vi "solar_voy Set VI Control.vi"(8 "error in (no error)":errorcluster, 11 "VI_SET_CONTROL":T1) -> (0 "error out":errorcluster)   [LabVIEW 2018]
doc: "This sets a VI control value by VI and Control name. The Value must be the LabVIEW native data type."
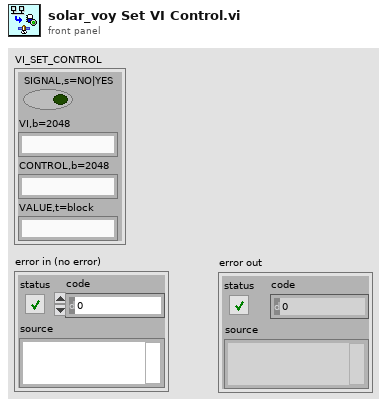
[diagram p1: front panel]
types:
  T1 = cluster{"SIGNAL,s=NO|YES":bool, "VI,b=2048":string, "CONTROL,b=2048":string, "VALUE,t=block":string}
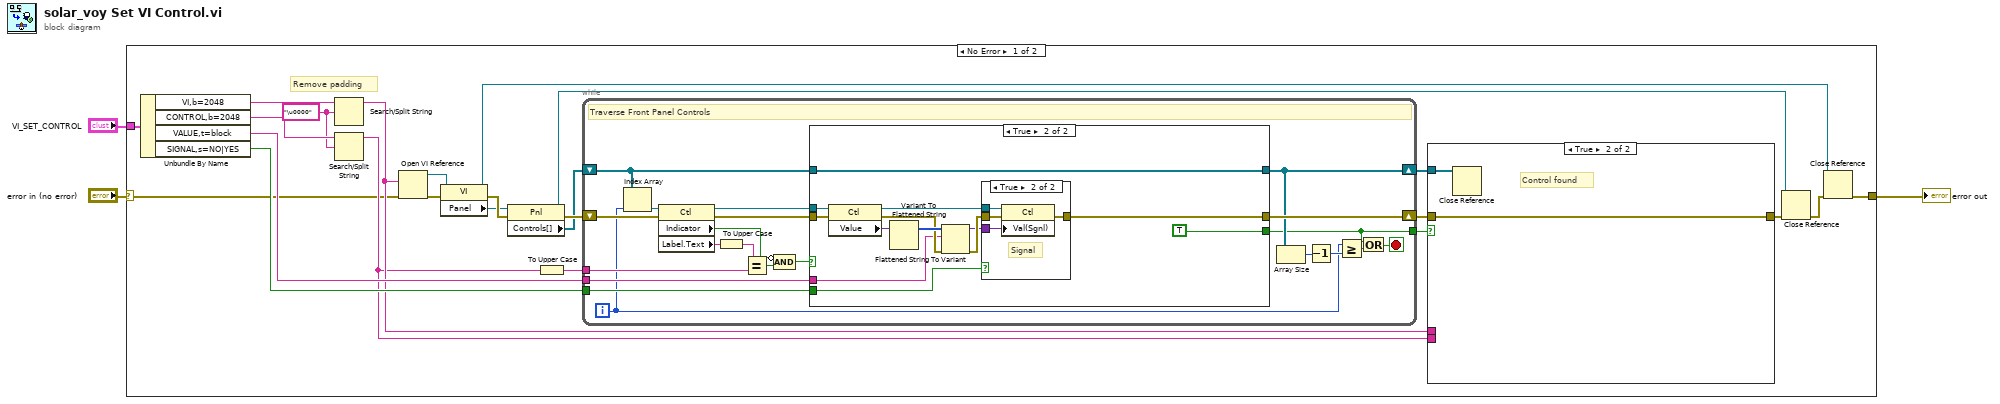
[diagram p0: block diagram]
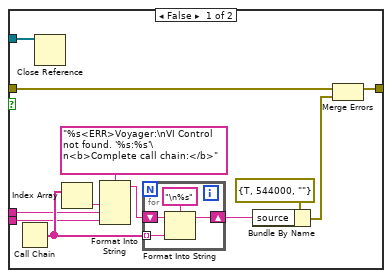
[diagram p2: hidden frame]
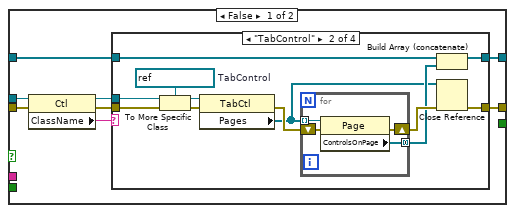
[diagram p3: hidden frame]
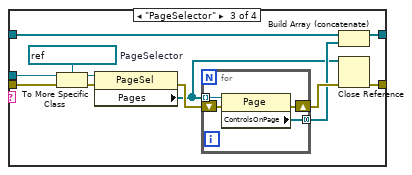
[diagram p5: hidden frame]
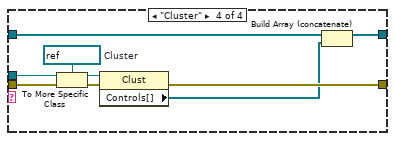
[diagram p6: hidden frame]
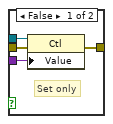
[diagram p7: hidden frame]
diagram:
  n1 = case shown="No Error" "error in (no error)" {
    selector: "error in (no error)" -> [w4 w139]
    tunnel: [w20 w139] -> w2
    tunnel: "VI_SET_CONTROL" -> [w5 _]
    frame No Error {
      w25 = "\u0000" ("search string/char (-)")
      # "Remove padding"
      n2 = Unbundle By Name(w5) -> ("VI,b=2048"=w27:string, "CONTROL,b=2048"=w26:string, "VALUE,t=block"=w22:string, "SIGNAL,s=NO|YES"=w19:bool)
      n3 = Search/Split String(string=w27, search string/char (-)=w25) -> (substring before match=w7:string)  [unwired: 1 in, 2 out]
      n4 = Search/Split String(string=w26, search string/char (-)=w25) -> (substring before match=w6:string)  [unwired: 1 in, 2 out]
      n5 = Open VI Reference(vi path=w7, error in (no error)=w4) -> (vi reference=w23:refnum<vi>, error out=w24:errorcluster)  [unwired: 4 in]
      n6 = property class="VI"(reference=w23, error in=w24) -> (reference out=w8:refnum<vi>, error out=w18:errorcluster, "Panel"=w17:refnum<vi>)
      n7 = property class="Pnl"(reference=w17, error in=w18) -> (reference out=w9:refnum<vi>, error out=w16:errorcluster, "Controls[]"=w15:refnum<vi>[])
      n8 = To Upper Case(1:w6) -> (0:w14:string)
      n9 = while {
        shift-right: [w57] -> w10
        shift-left: w16 -> [w66]
        shift-right: [w55] -> w13
        shift-left: w15 -> [w56]
        tunnel: w14 -> [w63]
        tunnel: w19 -> [w61]
        tunnel: w22 -> [w58]
        tunnel: [w49] -> w12
        i -> [w52]
        stop <- w50 stop-if-true
        # "Traverse Front Panel Controls"
        n10 = Index Array(array=w56, index=w52) -> (element=w65:refnum<vi>)
        n11 = property class="Ctl"(reference=w65, error in=w66) -> (reference out=w59:refnum<vi>, error out=w60:errorcluster, "Indicator"=w47:bool, "Label.Text"=w64:string)
        n12 = To Upper Case(1:w64) -> (0:w62:string)
        n13 = Equal?(x=w62, y=w63) -> (x = y?=w48:bool)
        n14 = Compound Arithmetic op=AND(invert w47, w48) -> (w46:bool)
        n15 = case shown="True" w46 {
          tunnel: w61 -> [_ w125]
          tunnel: w60 -> [w73 w130]
          tunnel: w59 -> [w71 w129]
          tunnel: w58 -> [_ w123]
          tunnel: [w69 w120] -> w57
          tunnel: [w68 w119] -> w55
          tunnel: w56 -> [w74 w119]
          tunnel: [_ TRUE] -> w49
          frame False {
            n16 = property class="Ctl"(reference=w71, error in=w73) -> (reference out=w70:refnum<vi>, error out=w72:errorcluster, "ClassName"=w67:string)
            n17 = case shown="\"TabControl\"" w67 {
              tunnel: w74 -> [w76 w88 w104 w117]
              tunnel: w72 -> [w75 w87 w103 w116]
              tunnel: w70 -> [_ w85 w101 w114]
              tunnel: [w75 w78 w94 w110] -> w69
              tunnel: [w76 w80 w96 w111] -> w68
              frame Default {
              }
              frame "TabControl" {
                w84 = refnum<vi> refnum  # TabControl
                n18 = To More Specific Class(target class=w84, reference=w85, error in=w87) -> (specific class reference=w82:refnum<vi>, error out=w86:errorcluster)
                n19 = property class="TabCtl"(reference=w82, error in=w86) -> (error out=w83:errorcluster, "Pages"=w77:refnum<vi>[])  [unwired: 1 out]
                n20 = for {
                  tunnel: w77 -> [w90] mode=indexing
                  shift-right: [w91] -> w81
                  shift-left: w83 -> [w92]
                  tunnel: [w89] -> w79 mode=concatenating
                  n21 = property class="Page"(reference=w90, error in=w92) -> (error out=w91:errorcluster, "ControlsOnPage"=w89:refnum<vi>[])  [unwired: 1 out]
                }
                n22 = Build Array (concatenate)(w88, w79) -> (w80:refnum<vi>[])
                n23 = Close Reference(reference=w77, error in (no error)=w81) -> (error out=w78:errorcluster)
              }
              frame "PageSelector" {
                w100 = refnum<vi> refnum  # PageSelector
                n24 = To More Specific Class(target class=w100, reference=w101, error in=w103) -> (specific class reference=w98:refnum<vi>, error out=w102:errorcluster)
                n25 = property class="PageSel"(reference=w98, error in=w102) -> (error out=w99:errorcluster, "Pages"=w93:refnum<vi>[])  [unwired: 1 out]
                n26 = for {
                  tunnel: w93 -> [w106] mode=indexing
                  shift-right: [w107] -> w97
                  shift-left: w99 -> [w108]
                  tunnel: [w105] -> w95 mode=concatenating
                  n27 = property class="Page"(reference=w106, error in=w108) -> (error out=w107:errorcluster, "ControlsOnPage"=w105:refnum<vi>[])  [unwired: 1 out]
                }
                n28 = Build Array (concatenate)(w104, w95) -> (w96:refnum<vi>[])
                n29 = Close Reference(reference=w93, error in (no error)=w97) -> (error out=w94:errorcluster)
              }
              frame "Cluster" {
                w113 = refnum<vi> refnum  # Cluster
                n30 = To More Specific Class(target class=w113, reference=w114, error in=w116) -> (specific class reference=w112:refnum<vi>, error out=w115:errorcluster)
                n31 = property class="Clust"(reference=w112, error in=w115) -> (error out=w110:errorcluster, "Controls[]"=w109:refnum<vi>[])  [unwired: 1 out]
                n32 = Build Array (concatenate)(w117, w109) -> (w111:refnum<vi>[])
              }
            }
          }
          frame True {
            n33 = property class="Ctl"(reference=w129, error in=w130) -> (reference out=w128:refnum<vi>, error out=w126:errorcluster, "Value"=w124:variant)
            n34 = Variant To Flattened String(Variant=w124) -> (1:w127:i16[])  [unwired: 1 out]
            n35 = Flattened String To Variant(4:w126, 6:w123, 7:w127) -> (0:w122:errorcluster, 3:w121:variant)
            n36 = case shown="True" w125 {
              tunnel: w122 -> [w134 w137]
              tunnel: w128 -> [w133 w138]
              tunnel: w121 -> [w132 w136]
              tunnel: [w131 w135] -> w120
              frame False {
                # "Set only"
                n37 = property class="Ctl"(reference=w133, error in=w134, "Value"=w132) -> (error out=w131:errorcluster)  [unwired: 1 out]
              }
              frame True {
                # "Signal"
                n38 = property class="Ctl"(reference=w138, error in=w137, "Val(Sgnl)"=w136) -> (error out=w135:errorcluster)  [unwired: 1 out]
              }
            }
          }
        }
        n39 = Array Size(array=w55) -> (size(s)=w54:i32)
        n40 = Decrement(x=w54) -> (x-1=w53:i32)
        n41 = Greater Or Equal?(x=w52, y=w53) -> (x >= y?=w51:bool)
        n42 = Or(x=w49, y=w51) -> (x .or. y?=w50:bool)
      }
      n43 = case shown="True" w12 {
        tunnel: w13 -> [w39 w45]
        tunnel: [w31 w44] -> w11
        tunnel: w10 -> [w32 w44]
        tunnel: w7 -> [w29 _]
        tunnel: w6 -> [w28 _]
        frame False {
          n44 = Call Chain() -> (call chain=w36:string[])
          n45 = Close Reference(reference=w39) -> ()  [unwired: 1 in, 1 out]
          n46 = Index Array(array=w36) -> (element=w34:string)  [unwired: 1 in]
          n47 = Format Into String(format string="%s<ERR>Voyager:\nVI Control not found. '%s:%s'\n<b>Complete call chain:</b>", w34, w29, w28) -> (resulting string=w35:string)  [unwired: 2 in, 1 out]
          n48 = for {
            tunnel: w36 -> [w43] mode=indexing
            shift-right: [w42] -> w37
            shift-left: w35 -> [w41]
            n49 = Format Into String(format string="\n%s", initial string=w41, w43) -> (resulting string=w42:string)  [unwired: 1 in, 1 out]
          }
          n50 = Bundle By Name(cluster=errorcluster {"status"=TRUE, "code"=544000, "source"=""} ("error in (no error)"), "source"=w37) -> (w30:errorcluster)
          n51 = Merge Errors(w32, w30) -> (w31:errorcluster)
        }
        frame True {
          # "Control found"
          n52 = Close Reference(reference=w45) -> ()  [unwired: 1 in, 1 out]
        }
      }
      n53 = Close Reference(reference=w9, error in (no error)=w11) -> (error out=w21:errorcluster)
      n54 = Close Reference(reference=w8, error in (no error)=w21) -> (error out=w20:errorcluster)
    }
    frame Error {
    }
  }
  "error out" <- w2
